vi "Next Recursively.vi"(8 "error in (no error)":errorcluster, 11 "LUnit Test Suite In":refnum<class "LUnit Test Suite.lvclass">) -> (0 "error out":errorcluster, 2 "Next Runnable":string, 3 "LUnit Test Suite Out":refnum<class "LUnit Test Suite.lvclass">)   [LabVIEW 2020, in "LUnit Test Suite.lvclass"]
uses:
  LUnit Test Suite.lvclass
  LUnit Test Suite.lvclass/LUnit Test Suite.ctl
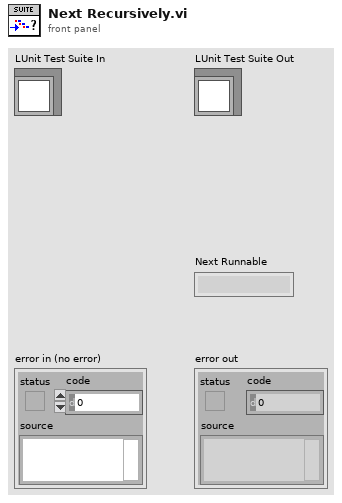
[diagram p1: front panel]
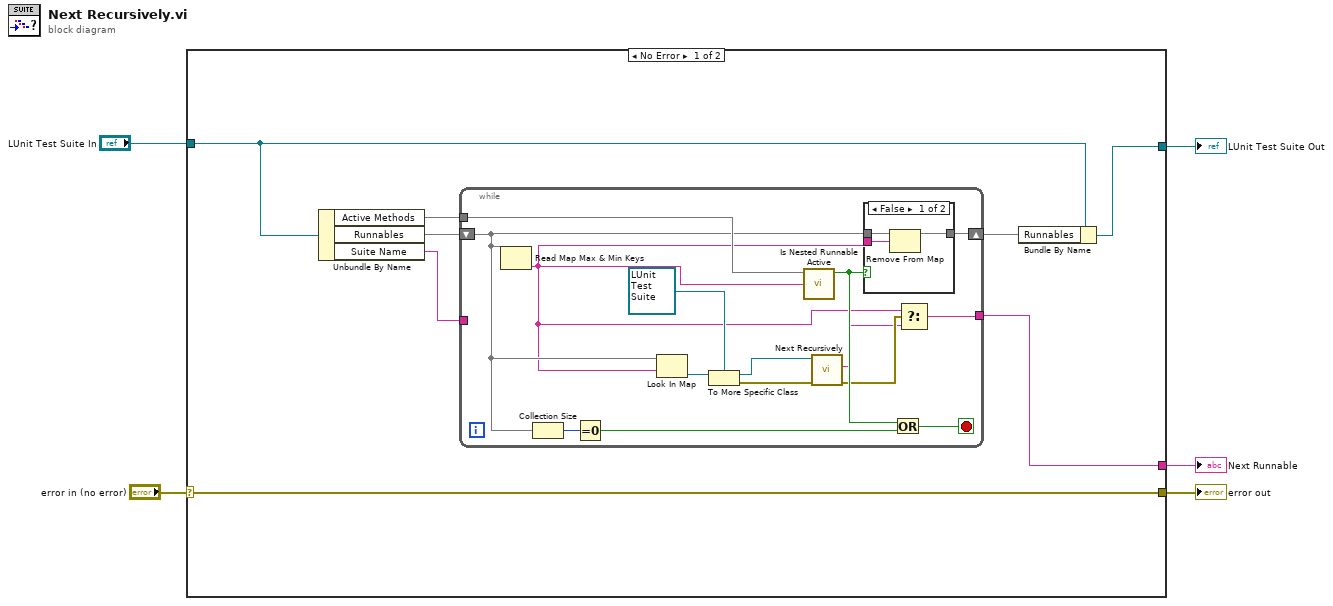
[diagram p0: block diagram]
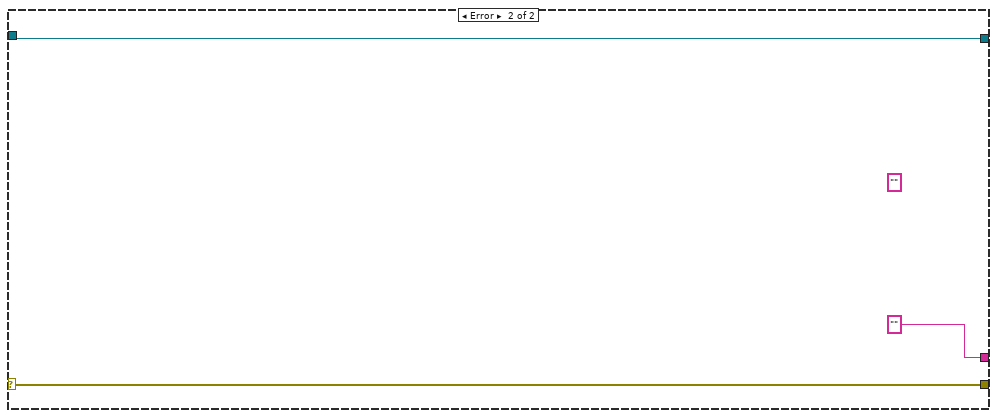
[diagram p3: hidden frame]
diagram:
  n1 = case shown="No Error" "error in (no error)" {
    selector: "error in (no error)" -> [w8 w34]
    tunnel: "LUnit Test Suite In" -> [w10 w35]
    tunnel: [w9 w35] -> w4
    tunnel: [w6 "" ("Suite Name")] -> w3
    tunnel: [w8 w34] -> w1
    frame No Error {
      n2 = Unbundle By Name(w10) -> ("Active Methods"=w12:set{string}, "Runnables"=w13:map{string, refnum<class "Runnable.lvclass">}, "Suite Name"=w7:string)
      n3 = while {
        tunnel: w12 -> [w28]
        shift-right: [w27] -> w11
        shift-left: w13 -> [w22]
        tunnel: w7 -> [_]
        tunnel: [w16] -> w6
        stop <- w26 stop-if-true
        n4 = Read Map Max & Min Keys(11:w22) -> (1:w15:string)  [unwired: 1 out]
        n5 = Collection Size(1:w22) -> (0:w25:i32)
        n6 = Equal To 0?(x=w25) -> (x = 0?=w24:bool)
        n7 = Look In Map(map=w22, key=w15) -> (value=w21:refnum<class "Runnable.lvclass">)  [unwired: 1 in, 1 out]
        n8 = To More Specific Class(target class=refnum<class "LUnit Test Suite.lvclass"> refnum ("LUnit Test Suite Out"), reference=w21) -> (specific class reference=w20:refnum<class "LUnit Test Suite.lvclass">, error out=w18:errorcluster)  [unwired: 1 in]
        n9 = call "Is Nested Runnable Active"("Name"=w15, "Active Methods"=w28) -> ("found?"=w23:bool)  [unwired: 9 in]
        n10 = call "Next Recursively.vi"("error in (no error)"=w18, "LUnit Test Suite In"=w20) -> ("error out"=w17:errorcluster, "Next Runnable"=w14:string)  [unwired: 7 in, 1 out]
        n11 = case shown="False" w23 {
          tunnel: w15 -> [w31 _]
          tunnel: [w30 w32] -> w27
          tunnel: w22 -> [w29 w32]
          frame False {
            n12 = Remove From Map(10:w31, 11:w29) -> (3:w30:map{string, refnum<class "Runnable.lvclass">})  [unwired: 2 out]
          }
          frame True {
          }
        }
        n13 = Or(x=w23, y=w24) -> (x .or. y?=w26:bool)
        n14 = Select(t=w15, s=w17, f=w14) -> (s? t:f=w16:string)
      }
      n15 = Bundle By Name(cluster=w10, "Runnables"=w11) -> (w9:refnum<class "LUnit Test Suite.lvclass">)
    }
    frame Error {
      (unwired) "" ("Name")
    }
  }
  "error out" <- w1
  "LUnit Test Suite Out" <- w4
  "Next Runnable" <- w3
